vi "Resideo Parse Data.vi"(8 "error in (no error)":errorcluster, 10 "LDO Data":u16[](array[numeric]), 11 "Vesta Data 1":u16[](array[numeric])) -> (0 "error out":errorcluster, 3 "Vesta Data Output":T1)   [LabVIEW 2020]
uses:
  Type Definitions/Vesta Info.ctl
panel:
  in  "Vesta Data":T1
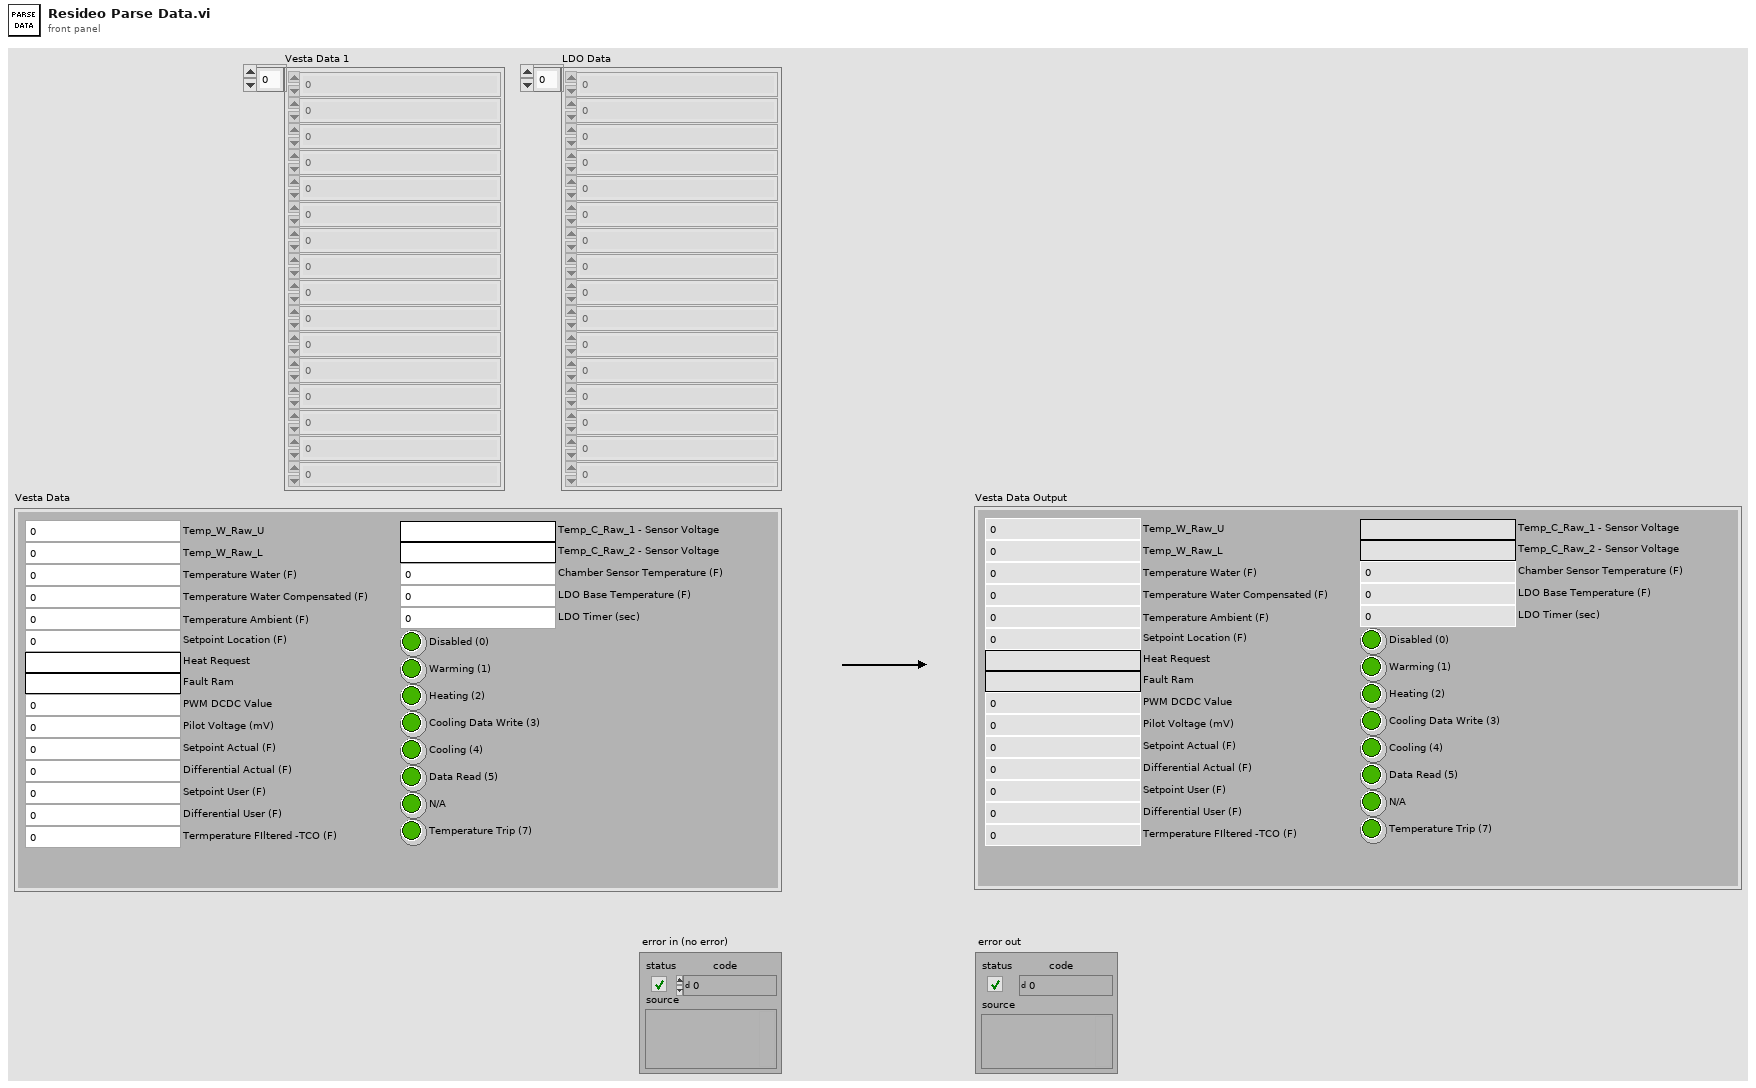
[diagram p1: front panel]
types:
  T1 = typedef "Vesta Info.ctl" = cluster{"Temp_W_Raw_U":u16, "Temp_W_Raw_L":u16, "Temperature Water (F)":dbl, "Temperature Water Compensated (F)":dbl, "Temperature Ambient (F)":dbl, "Setpoint Location (F)":dbl, "Heat Request":string, "Fault Ram":string, "PWM DCDC Value":u16, "Pilot Voltage (mV)":dbl, "Setpoint Actual (F)":dbl, "Differential Actual (F)":dbl, "Setpoint User (F)":dbl, "Differential User (F)":dbl, "Termperature FIltered -TCO (F)":dbl, "Temp_C_Raw_1 - Sensor Voltage":string, "Temp_C_Raw_2 - Sensor Voltage":string, "Chamber Sensor Temperature (F)":dbl, "LDO Base Temperature (F)":dbl, "LDO Timer (sec)":i16, "Disabled (0)":bool, "Warming (1)":bool, "Heating (2)":bool, "Cooling Data Write (3)":bool, "Cooling (4)":bool, "Data Read (5)":bool, "N/A":bool, "Temperature Trip (7)":bool}
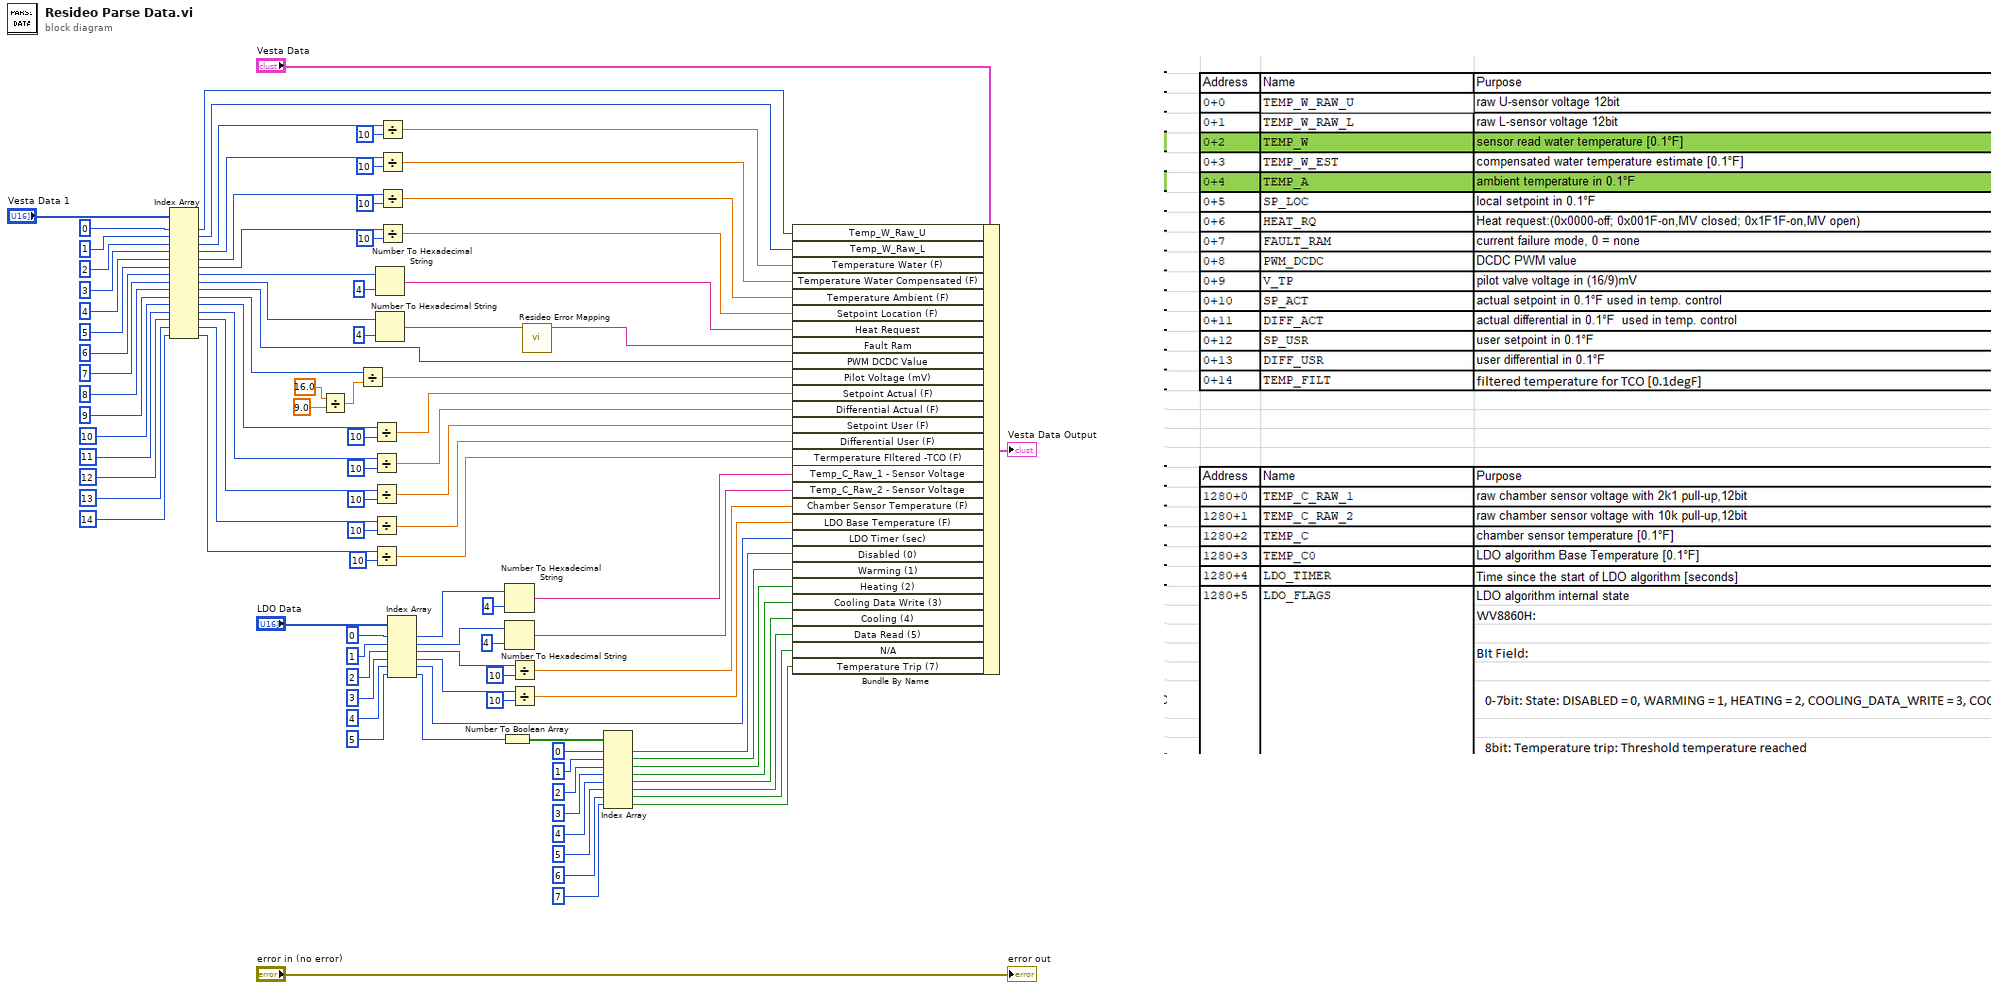
[diagram p0: block diagram]
diagram:
  n1 = Index Array(array="Vesta Data 1", index #1=0 ("index"), index #2=1 ("index"), index #3=2 ("index"), index #4=3 ("index"), index #5=4 ("index"), index #6=5 ("index"), index #7=6 ("index"), index #8=7 ("index"), index #9=8 ("index"), index #10=9 ("index"), index #11=10 ("index"), index #12=11 ("index"), index #13=12 ("index"), index #14=13 ("index"), index #15=14 ("index")) -> (element #1=w94:u16, element #2=w93:u16, element #3=w91:u16, element #4=w87:u16, element #5=w83:u16, element #6=w78:u16, element #7=w75:u16, element #8=w71:u16, element #9=w68:u16, element #10=w64:u16, element #11=w59:u16, element #12=w55:u16, element #13=w50:u16, element #14=w46:u16, element #15=w42:u16)
  n2 = Divide(x=16.0, y=9.0) -> (x/y=w63:dbl)
  n3 = Divide(x=w64, y=w63) -> (x/y=w62:dbl)
  n4 = Divide(x=w59, y=u16 10) -> (x/y=w58:dbl)
  n5 = Divide(x=w55, y=u16 10) -> (x/y=w54:dbl)
  n6 = Divide(x=w50, y=u16 10) -> (x/y=w49:dbl)
  n7 = Divide(x=w46, y=u16 10) -> (x/y=w45:dbl)
  n8 = Divide(x=w42, y=u16 10) -> (x/y=w41:dbl)
  n9 = Number To Hexadecimal String(1:i16 4 ("width (-)"), 2:w75) -> (0:w74:string)
  n10 = Number To Hexadecimal String(1:i16 4 ("width (-)"), 2:w71) -> (0:w70:string)
  n11 = Divide(x=w91, y=u16 10) -> (x/y=w90:dbl)
  n12 = Divide(x=w87, y=u16 10) -> (x/y=w86:dbl)
  n13 = Divide(x=w83, y=u16 10) -> (x/y=w81:dbl)
  n14 = Divide(x=w78, y=u16 10) -> (x/y=w77:dbl)
  n15 = Index Array(array="LDO Data", index #1=0 ("index"), index #2=1 ("index"), index #3=2 ("index"), index #4=3 ("index"), index #5=4 ("index"), index #6=5 ("index")) -> (element #1=w37:u16, element #2=w33:u16, element #3=w29:u16, element #4=w25:u16, element #5=w22:u16, element #6=w20:u16)
  n16 = Number To Boolean Array(number=w20) -> (Boolean array=w19:bool[])
  n17 = Number To Hexadecimal String(1:i16 4 ("width (-)"), 2:w37) -> (0:w36:string)
  n18 = Number To Hexadecimal String(1:i16 4 ("width (-)"), 2:w33) -> (0:w32:string)
  n19 = Divide(x=w29, y=u16 10) -> (x/y=w28:dbl)
  n20 = Divide(x=w25, y=u16 10) -> (x/y=w24:dbl)
  n21 = call "Resideo Error Mapping.vi"("Error Code Number"=w70) -> ("Error Status"=w1:string)  [unwired: 10 in]
  n22 = Index Array(array=w19, index #1=0 ("index"), index #2=1 ("index"), index #3=2 ("index"), index #4=3 ("index"), index #5=4 ("index"), index #6=5 ("index"), index #7=6 ("index"), index #8=7 ("index")) -> (element #1=w10:bool, element #2=w9:bool, element #3=w8:bool, element #4=w7:bool, element #5=w6:bool, element #6=w5:bool, element #7=w4:bool, element #8=w3:bool)
  n23 = Bundle By Name(cluster="Vesta Data", "Temp_W_Raw_U"=w94, "Temp_W_Raw_L"=w93, "Temperature Water (F)"=w90, "Temperature Water Compensated (F)"=w86, "Temperature Ambient (F)"=w81, "Setpoint Location (F)"=w77, "Heat Request"=w74, "Fault Ram"=w1, "PWM DCDC Value"=w68, "Pilot Voltage (mV)"=w62, "Setpoint Actual (F)"=w58, "Differential Actual (F)"=w54, "Setpoint User (F)"=w49, "Differential User (F)"=w45, "Termperature FIltered -TCO (F)"=w41, "Temp_C_Raw_1 - Sensor Voltage"=w36, "Temp_C_Raw_2 - Sensor Voltage"=w32, "Chamber Sensor Temperature (F)"=w28, "LDO Base Temperature (F)"=w24, "LDO Timer (sec)"=w22, "Disabled (0)"=w10, "Warming (1)"=w9, "Heating (2)"=w8, "Cooling Data Write (3)"=w7, "Cooling (4)"=w6, "Data Read (5)"=w5, "N/A"=w4, "Temperature Trip (7)"=w3) -> (→"Vesta Data Output":T1)
  "error out" <- "error in (no error)"
